vi "SUB_SFCS_SendResult_CtlMCS.vi"(1 "MCS_Server_enable?":bool, 2 "ErrorCode":string, 3 "PASS_Fail (1/0)":i8) -> (0 "Sent OK ?":bool)   [LabVIEW 2011]
uses:
  Instance           8 34Saved   SUB_SFCS_SendResult_CtlMCS .vi
  Instance           7 34Saved   SUB_SFCS_SendResult_CtlMCS .vi
  Instance           4 34Saved   SUB_SFCS_SendResult_CtlMCS .vi
  Instance          10 34Saved   SUB_SFCS_SendResult_CtlMCS .vi
  Instance          11 34Saved   SUB_SFCS_SendResult_CtlMCS .vi
  data/MCSDLL.dll
  Instance          14 34Saved   SUB_SFCS_SendResult_CtlMCS .vi
  Instance          15 34Saved   SUB_SFCS_SendResult_CtlMCS .vi
panel:
  out "output param":string
  out "SFCS System Enable":string
  out "OperatorID":string
  out "Line":string
  out "SN":string
  out "Station":string
  out "STAGE":string
  out "SFCS_IP":string
  in  "URL":string
  # "Send Result SFCS_Complete"
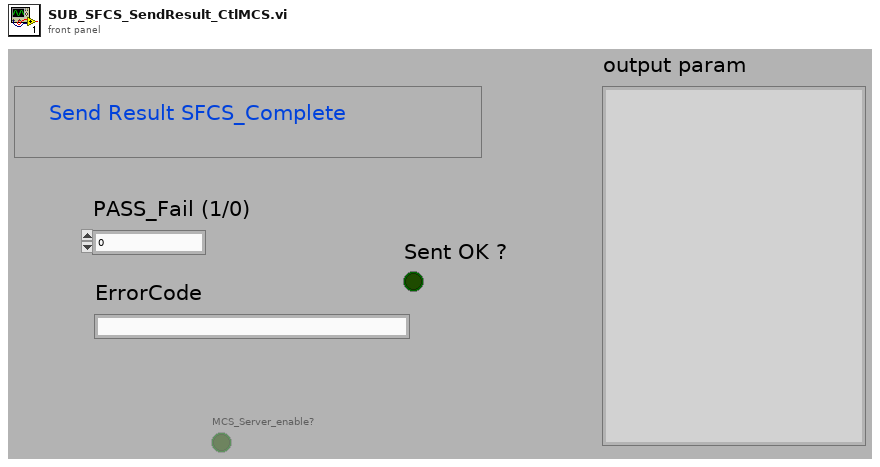
[diagram p1: front panel]
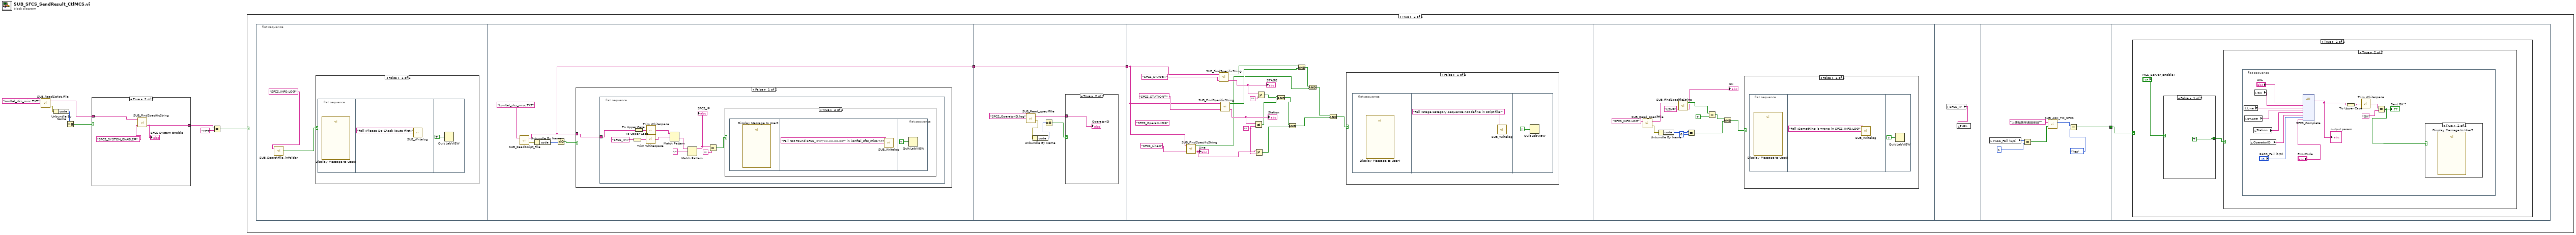
[diagram p0: block diagram]
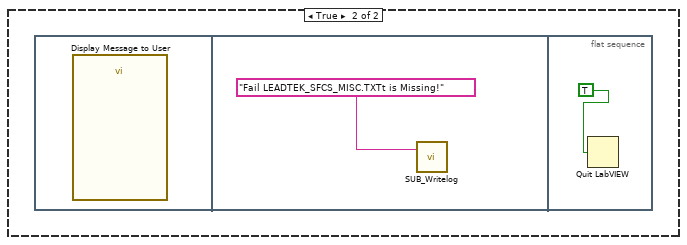
[diagram p5: hidden frame]
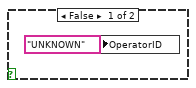
[diagram p6: hidden frame]
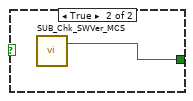
[diagram p10: hidden frame]
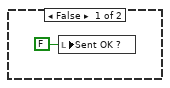
[diagram p11: hidden frame]
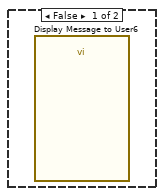
[diagram p12: hidden frame]
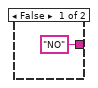
[diagram p13: hidden frame]
diagram:
  n1 = call "SUB_ReadScript_File.vi"("Script FileName"="konftel_sfcs_misc.TXT") -> ("error out"=w8:errorcluster, "text"=w2:string)  [unwired: 1 in]
  n2 = Unbundle By Name(w8) -> ("code"=w7:i32)
  n3 = Equal To 0?(x=w7) -> (x = 0?=w6:bool)
  n4 = case shown="True" w6 {
    tunnel: w2 -> [_ w12]
    tunnel: ["NO" ("before \"; \" string") w10] -> w4
    frame False {
    }
    frame True {
      n5 = call "SUB_FindSpecificString.vi"("Find this String"="SFCS_SYSTEM_ENABLE=", "String data"=w12) -> ("before \"; \" string"=w10:string)  [unwired: 2 in, 1 out]
      "SFCS System Enable" <- w10
    }
  }
  n6 = Equal?(x=w4, y="YES") -> (x = y?=w5:bool)
  n7 = case shown="True" w5 {
    frame False {
    }
    frame True {
      n8 = flat-sequence {
        tunnel: [w21] -> w14
        tunnel: w14 -> [w46]
        tunnel: [w46] -> w13
        tunnel: w13 -> [w64]
        tunnel: [w89] -> w15
        tunnel: w15 -> [w93]
        frame #0 {
          n9 = call "SUB_SearchFile_inFolder.vi"("Search Filename in Folder"="SFCS_INFO.LOG") -> ("File Existing True/Flase"=w16:bool)  [unwired: 1 in]
          n10 = case shown="False" w16 {
            frame False {
              n11 = flat-sequence {
                frame #0 {
                  n12 = call "Display Message to User3"() -> ()  [unwired: 10 in, 2 out]
                }
                frame #1 {
                  n13 = call "SUB_Writelog.vi"("Pass/Fail"="Fail :Please Do Check Route First !") -> ()  [unwired: 2 in]
                }
                frame #2 {
                  n14 = Quit LabVIEW(quit? (T)=TRUE) -> ()
                }
              }
            }
            frame True {
            }
          }
        }
        frame #1 {
          n15 = call "SUB_ReadScript_File.vi"("Script FileName"="konftel_sfcs_misc.TXT") -> ("error out"=w24:errorcluster, "text"=w21:string)  [unwired: 1 in]
          n16 = Unbundle By Name(w24) -> ("code"=w23:i32)
          n17 = Not Equal To 0?(x=w23) -> (x != 0?=w22:bool)
          n18 = case shown="False" w22 {
            tunnel: w21 -> [w25 _]
            frame False {
              n19 = flat-sequence {
                tunnel: w25 -> [w31]
                frame #0 {
                  n20 = To Upper Case(1:"SFCS_IP=" ("string")) -> (0:w35:string)
                  n21 = To Upper Case(1:w31) -> (0:w36:string)
                  n22 = call <vilib>:"Trim Whitespace.vi"("string"=w35) -> ("trimmed string"=w33:string)  [unwired: 1 in]
                  n23 = call <vilib>:"Trim Whitespace.vi"("string"=w36) -> ("trimmed string"=w32:string)  [unwired: 1 in]
                  n24 = Match Pattern(string=w32, regular expression=w33) -> (after substring=w30:string)  [unwired: 1 in, 3 out]
                  n25 = Match Pattern(string=w30, regular expression=";") -> (before substring=w28:string)  [unwired: 1 in, 3 out]
                  "SFCS_IP" <- w28
                  n26 = Equal?(x=w28, y="") -> (x = y?=w26:bool)
                  n27 = case shown="True" w26 {
                    frame False {
                    }
                    frame True {
                      n28 = flat-sequence {
                        frame #0 {
                          n29 = call "Display Message to User2"() -> ()  [unwired: 10 in, 2 out]
                        }
                        frame #1 {
                          n30 = call "SUB_Writelog.vi"("Pass/Fail"="Fail Not Found SFCS_IP=\"xx.xx.xx.xx\" in konftel_sfcs_misc.TXT !") -> ()  [unwired: 2 in]
                        }
                        frame #2 {
                          n31 = Quit LabVIEW(quit? (T)=TRUE) -> ()
                        }
                      }
                    }
                  }
                }
              }
            }
            frame True {
              n32 = flat-sequence {
                frame #0 {
                  n33 = call "Display Message to User"() -> ()  [unwired: 10 in, 2 out]
                }
                frame #1 {
                  n34 = call "SUB_Writelog.vi"("Pass/Fail"="Fail LEADTEK_SFCS_MISC.TXTt is Missing!") -> ()  [unwired: 2 in]
                }
                frame #2 {
                  n35 = Quit LabVIEW(quit? (T)=TRUE) -> ()
                }
              }
            }
          }
        }
        frame #2 {
          n36 = call "SUB_Read_specifFile.vi"("name or relative path"="SFCS_OperatorID.log") -> ("error out"=w44:errorcluster, "text"=w41:string)  [unwired: 1 in]
          n37 = Unbundle By Name(w44) -> ("code"=w43:i32)
          n38 = Equal To 0?(x=w43) -> (x = 0?=w42:bool)
          n39 = case shown="True" w42 {
            tunnel: w41 -> [_ w48]
            frame False {
              n40 = local write "OperatorID"("UNKNOWN" ("OperatorID")) -> ()
            }
            frame True {
              "OperatorID" <- w48
            }
          }
        }
        frame #3 {
          (unwired) "SFCS_OperatorID="
          w59 = ""
          n41 = call "SUB_FindSpecificString.vi"("Find this String"="SFCS_Line=", "String data"=w64) -> ("before \"; \" string"=w60:string, "Found"=w50:bool)  [unwired: 2 in]
          "Line" <- w60
          n42 = call "SUB_FindSpecificString.vi"("Find this String"="SFCS_STAGE=" ("string"), "String data"=w64) -> ("before \"; \" string"=w62:string, "Found"=w55:bool)  [unwired: 2 in]
          "STAGE" <- w62
          n43 = call "SUB_FindSpecificString.vi"("Find this String"="SFCS_STATION=" ("string"), "String data"=w64) -> ("before \"; \" string"=w61:string, "Found"=w54:bool)  [unwired: 2 in]
          "Station" <- w61
          n44 = Not Equal?(x=w61, y=w59) -> (x != y?=w57:bool)
          n45 = Not Equal?(x=w60, y=w59) -> (x != y?=w49:bool)
          n46 = Not Equal?(x=w62, y="") -> (x != y?=w58:bool)
          n47 = And(x=w58, y=w57) -> (x .and. y?=w56:bool)
          n48 = And(x=w56, y=w49) -> (x .and. y?=w51:bool)
          n49 = And(x=w55, y=w54) -> (x .and. y?=w53:bool)
          n50 = And(x=w53, y=w50) -> (x .and. y?=w52:bool)
          n51 = And(x=w52, y=w51) -> (x .and. y?=w67:bool)
          n52 = case shown="False" w67 {
            frame False {
              n53 = flat-sequence {
                frame #0 {
                  n54 = call "Display Message to User4"() -> ()  [unwired: 10 in, 2 out]
                }
                frame #1 {
                  n55 = call "SUB_Writelog.vi"("Pass/Fail"="Fail :Stage,Category,Sequence not define in script file!") -> ()  [unwired: 2 in]
                }
                frame #2 {
                  n56 = Quit LabVIEW(quit? (T)=TRUE) -> ()
                }
              }
            }
            frame True {
            }
          }
        }
        frame #4 {
          n57 = call "SUB_Read_specifFile.vi"("name or relative path"="SFCS_INFO.LOG") -> ("error out"=w81:errorcluster, "text"=w80:string)  [unwired: 1 in]
          n58 = Unbundle By Name(w81) -> ("code"=w78:i32)
          n59 = call "SUB_FindSpecificString.vi"("Find this String"="USN=", "String data"=w80) -> ("before \"; \" string"=→"SN":string, "Found"=w76:bool)  [unwired: 2 in]
          n60 = Equal?(x=w78, y=0) -> (x = y?=w73:bool)
          n61 = Equal?(x=w76, y=TRUE) -> (x = y?=w74:bool)
          n62 = And(x=w74, y=w73) -> (x .and. y?=w71:bool)
          n63 = case shown="False" w71 {
            frame False {
              n64 = flat-sequence {
                frame #0 {
                  n65 = call "Display Message to User5"() -> ()  [unwired: 10 in, 2 out]
                }
                frame #1 {
                  n66 = call "SUB_Writelog.vi"("Pass/Fail"="Fail :Something is wrong in SFCS_INFO.LOG") -> ()  [unwired: 2 in]
                }
                frame #2 {
                  n67 = Quit LabVIEW(quit? (T)=TRUE) -> ()
                }
              }
            }
            frame True {
            }
          }
        }
        frame #5 {
          n68 = local read "SFCS_IP"() -> (w85:string)
          n69 = local write "URL"(w85) -> ()
        }
        frame #6 {
          n70 = local read "PASS_Fail (1/0)"() -> (w88:i8)
          n71 = Equal?(x=w88, y=i8 1) -> (x = y?=w86:bool)
          n72 = call "SUB_ASK_TO_SFCS.vi"("測試結果(報告)"=w86, "Question:"="上傳結果至遠端係統?") -> ("yes/no"=w91:enum32{"No Selection", "Yes", "No", "None"})  [unwired: 1 in]
          n73 = Equal?(x=w91, y=enum32{"No Selection", "Yes", "No", "None"}."Yes") -> (x = y?=w89:bool)
        }
        frame #7 {
          n74 = case shown="True" w93 {
            frame False {
            }
            frame True {
              n75 = case shown="False" "MCS_Server_enable?" {
                tunnel: [TRUE w97] -> w94
                frame False {
                }
                frame True {
                  n76 = call "SUB_Chk_SWVer_MCS.vi"() -> ("OK ?"=w97:bool)  [unwired: 2 in, 1 out]
                }
              }
              n77 = case shown="True" w94 {
                frame False {
                  n78 = local write "Sent OK ?"(FALSE ("Sent OK ?")) -> ()
                }
                frame True {
                  n79 = flat-sequence {
                    frame #0 {
                      n80 = local read "Line"() -> (w109:string)
                      n81 = local read "STAGE"() -> (w108:string)
                      n82 = local read "OperatorID"() -> (w106:string)
                      n83 = local read "Station"() -> (w107:string)
                      n84 = local read "SN"() -> (w110:string)
                      n85 = dll-call lib="D:/S8300E_Project/data/MCSDLL.dll" fn="SFCS_Complete"("URL"="URL", "SN"=w110, "Line"=w109, "Stage"=w108, "Station"=w107, "OperatorID"=w106, "PASS_Fail"="PASS_Fail (1/0)", "ErrorCode"="ErrorCode") -> (w103:string)  [unwired: 11 in, 2 out]
                      "output param" <- w103
                      n86 = To Upper Case(1:w103) -> (0:w104:string)
                      n87 = call <vilib>:"Trim Whitespace.vi"("string"=w104) -> ("trimmed string"=w102:string)  [unwired: 1 in]
                      n88 = Equal?(x=w102, y="OK") -> (x = y?=w100:bool)
                      "Sent OK ?" <- w100
                      n89 = case shown="True" w100 {
                        frame False {
                          n90 = call "Display Message to User6"() -> ()  [unwired: 10 in, 2 out]
                        }
                        frame True {
                          n91 = call "Display Message to User7"() -> ()  [unwired: 10 in, 2 out]
                        }
                      }
                    }
                  }
                }
              }
            }
          }
        }
      }
    }
  }
